vi "MovingAverage.vi"(9 "Moving Average interval":i32, 11 "Input Array":dbl[](array[numeric])) -> (2 "M.A. Array":dbl[](array[numeric]))   [LabVIEW 2017]
uses:
  <vilib>/Analysis/3filter.llb/FIR Filter (DBL).vi
  <vilib>/Analysis/NI_AALBase.lvlib
panel:
  out "Target Index (L)":i32=6
  out "Pav (Pa)":dbl=-49199.19854911039 format="%0.4e"
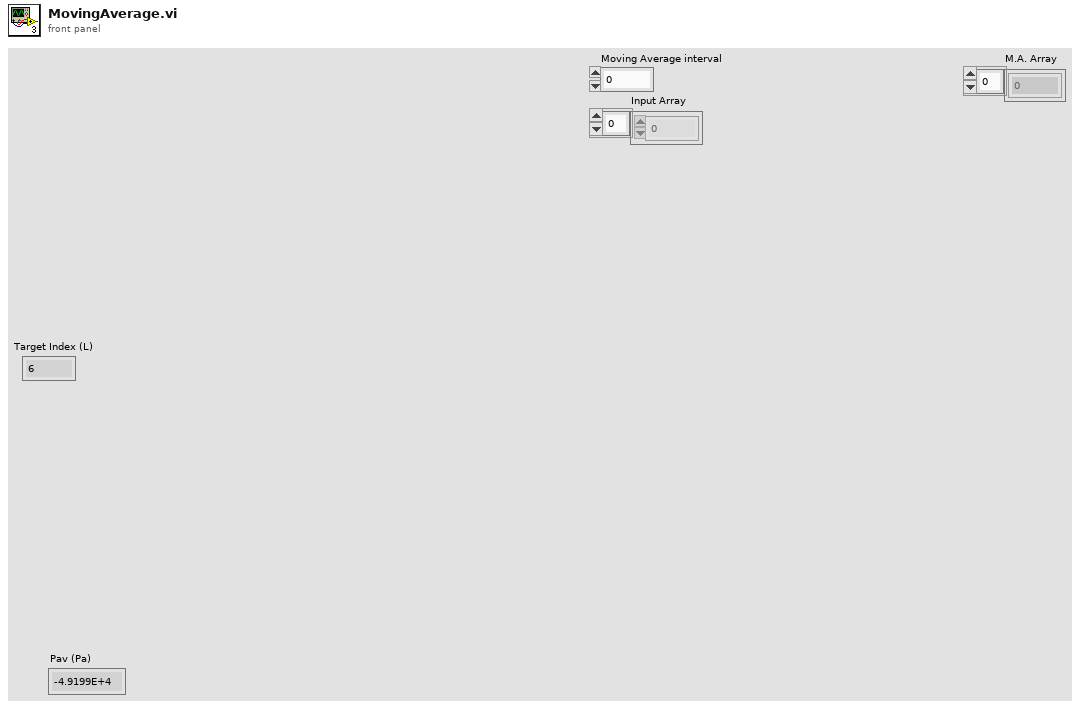
[diagram p1: front panel]
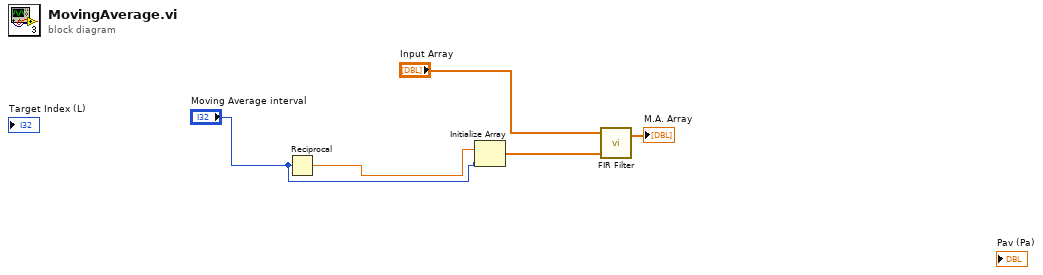
[diagram p0: block diagram]
diagram:
  n1 = Reciprocal(x="Moving Average interval") -> (1/x=w5:dbl)
  n2 = Initialize Array(w5, "Moving Average interval") -> (w4:dbl[])
  n3 = call-poly <vilib>:"FIR Filter.vi"("FIR Coefficients"=w4, "X"="Input Array") -> ("Filtered X"=→"M.A. Array":dbl[])  [unwired: 2 in, 1 out]
